vi "Remove Object.vi"(8 "error in (no error)":errorcluster, 10 "UUID":string, 11 "Controller in":refnum<class "Controller.lvclass">) -> (0 "error out":errorcluster, 3 "Controller out":refnum<class "Controller.lvclass">)   [LabVIEW 2013, in "SET Project Editor.lvlib" / "Controller.lvclass"]
uses:
  Controller.lvclass
  Controller.lvclass/Controller.ctl
  SET Project Data/Project Data Class/Project Data.lvclass
  SET Project Data/Menu Class/Menu Data.lvclass/Menu Data.ctl
  SET Project Data/VI Class/VI Data.lvclass
  SET Project Data/Control Classes/GObject/GObject.lvclass/GObject.ctl
  <vilib>/ActorFramework/Message Enqueuer/Message Enqueuer.lvclass/Message Enqueuer.ctl
  SET Project Data/Menu Class/Write Menu Item LUT.vi
  SET Project Data/Menu Class/Read Menu Item LUT.vi
  SET Project Data/Control Classes/GObject/Write Items.vi
  SET Project Data/Control Classes/GObject/Read Items.vi
  <vilib>/ActorFramework/Message Enqueuer/Enqueue.vi
  <vilib>/ActorFramework/Message Priority Queue/Priority Enqueue.vi
  UI View Messages/UI Refresh Data Msg/UI Refresh Data Msg.lvclass
  SET Project Editor.lvlib
  SET Project Data/Control Classes/GObject/GObject.lvclass
  SET Project Data/Menu Class/Menu Data.lvclass
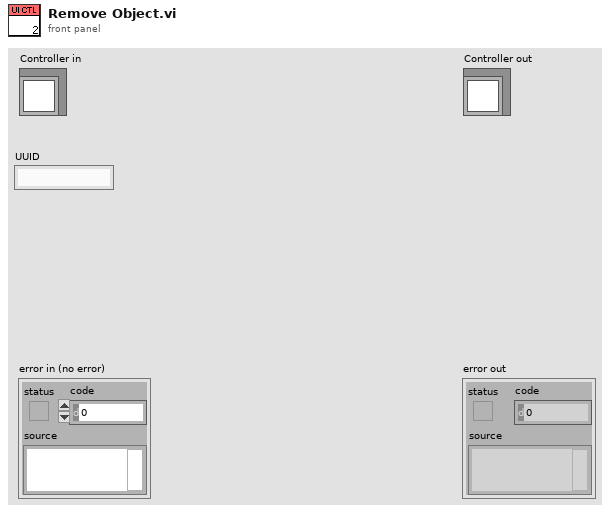
[diagram p1: front panel]
types:
  T1 = typedef "SET Project Editor.lvlib/UID Types.ctl" = enum16{"Invalid", "VI File", "GObject", "GObject Item", "RTM File", "RTM Item"}
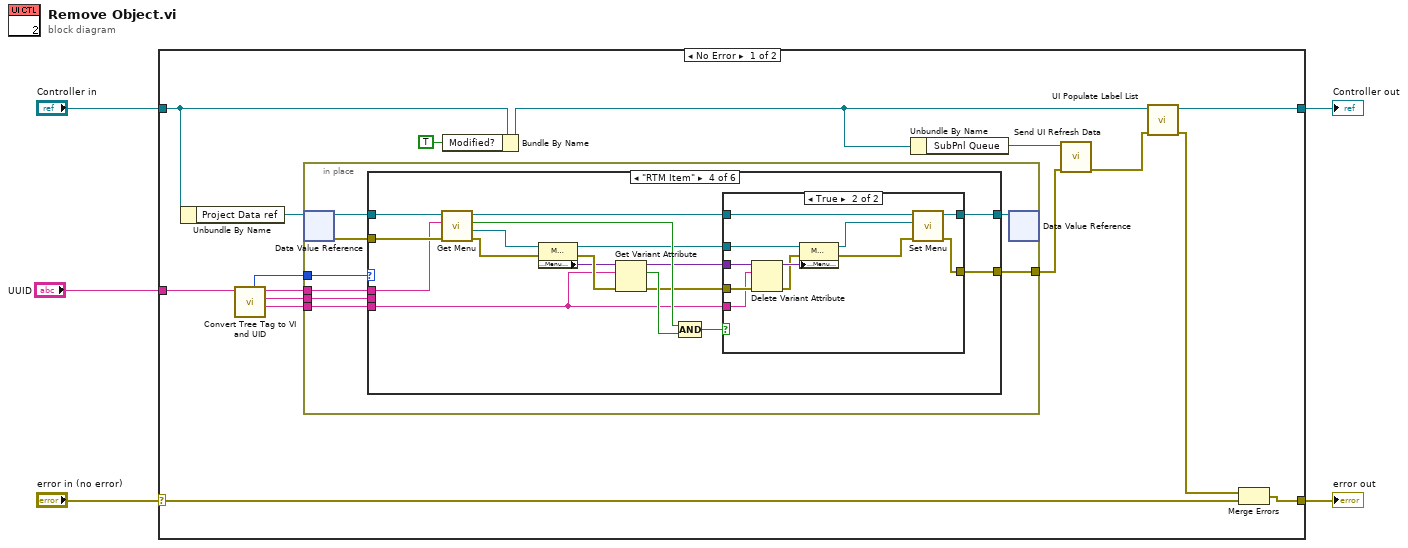
[diagram p0: block diagram]
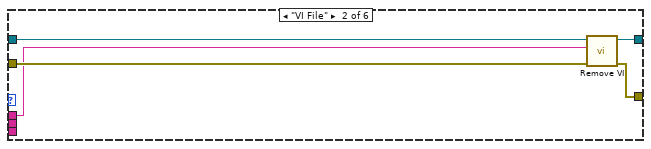
[diagram p3: hidden frame]
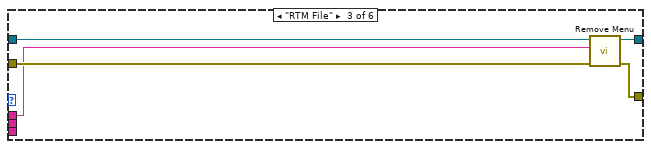
[diagram p4: hidden frame]
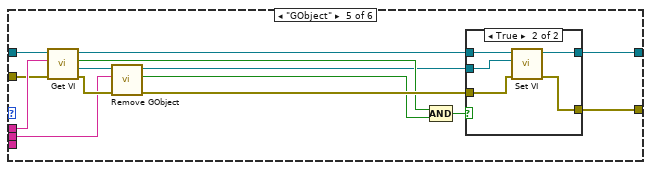
[diagram p6: hidden frame]
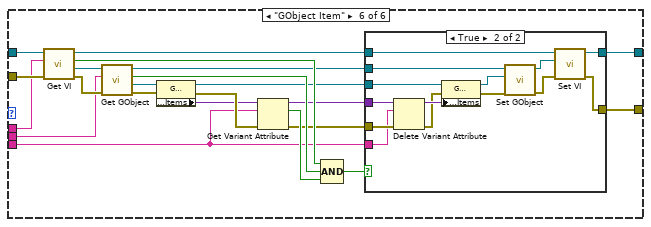
[diagram p8: hidden frame]
diagram:
  n1 = case shown="No Error" "error in (no error)" {
    selector: "error in (no error)" -> [w20 w132]
    tunnel: [w19 w132] -> w4
    tunnel: [w13 w131] -> w2
    tunnel: "Controller in" -> [w16 w131]
    tunnel: "UUID" -> [w10 _]
    frame No Error {
      n2 = Unbundle By Name(w16) -> ("Project Data ref"=w21:refnum<data-value>)
      n3 = call "Convert Tree Tag to VI and UID.vi"("Tree Tag"=w10) -> ("Item Name"=w6:string, "GObject UID"=w7:string, "File Path (Relative)"=w8:string, "UID Type"=w9:T1)  [unwired: 7 in]
      n4 = in-place {
        in-place-border: [w28] -> w17
        in-place-border: w9 -> [w25]
        in-place-border: w8 -> [w24]
        in-place-border: w7 -> [w23]
        in-place-border: w6 -> [w22]
        n5 = in-place-dvr #1(w21) -> (w27:refnum<class "Project Data.lvclass">, w26:errorcluster)
        n6 = case shown="\"RTM Item\"" w25 {
          tunnel: [w31 w35 w40 w46 w76 w97] -> w29
          tunnel: [w30 w33 w38 w42 w73 w96] -> w28
          tunnel: w27 -> [w31 w36 w41 w47 w77 w99]
          tunnel: w26 -> [w30 w34 w39 w45 w74 w98]
          tunnel: w24 -> [_ w32 w37 w44 w75 w95]
          tunnel: w23 -> [_ _ _ _ w72 w94]
          tunnel: w22 -> [_ _ _ w43 _ w93]
          frame "Invalid", Default {
          }
          frame "VI File" {
            n7 = call "Remove VI.vi"("error in (no error)"=w34, "VI Name"=w32, "ProjectData in"=w36) -> ("error out"=w33:errorcluster, "ProjectData out"=w35:refnum<class "Project Data.lvclass">)  [unwired: 5 in, 2 out]
          }
          frame "RTM File" {
            n8 = call "Remove Menu.vi"("error in (no error)"=w39, "Menu Name"=w37, "ProjectData in"=w41) -> ("error out"=w38:errorcluster, "ProjectData out"=w40:refnum<class "Project Data.lvclass">)  [unwired: 5 in, 2 out]
          }
          frame "RTM Item" {
            n9 = call-dynamic "Get Menu.vi"("error in (no error)"=w45, "Menu Path (Relative)"=w44, "ProjectData in"=w47) -> ("error out"=w58:errorcluster, "Menu Data out"=w57:refnum<class "Menu Data.lvclass">, "found"=w54:bool, "ProjectData out"=w48:refnum<class "Project Data.lvclass">)  [unwired: 5 in]
            n10 = property class="Menu Data.lvclass"(reference=w57, error in=w58) -> (reference out=w49:refnum<class "Menu Data.lvclass">, error out=w53:errorcluster, "Properties:Menu Item LUT"=w50:variant)
            n11 = Get Variant Attribute(Variant=w50, name=w43, error in=w53) -> (duplicate Variant=w51:variant, found=w55:bool, error out=w52:errorcluster)  [unwired: 1 in, 1 out]
            n12 = Compound Arithmetic op=AND(w54, w55) -> (w56:bool)
            n13 = case shown="True" w56 {
              tunnel: w48 -> [w60 w71]
              tunnel: [w60 w70] -> w46
              tunnel: w49 -> [_ w68]
              tunnel: [w59 w67] -> w42
              tunnel: w51 -> [_ w65]
              tunnel: w52 -> [w59 w64]
              tunnel: w43 -> [_ w63]
              frame False {
              }
              frame True {
                n14 = Delete Variant Attribute(4:w64, 6:w63, 7:w65) -> (0:w66:errorcluster, 3:w69:variant)  [unwired: 1 out]
                n15 = property class="Menu Data.lvclass"(reference=w68, error in=w66, "Properties:Menu Item LUT"=w69) -> (reference out=w62:refnum<class "Menu Data.lvclass">, error out=w61:errorcluster)
                n16 = call-dynamic "Set Menu.vi"("error in (no error)"=w61, "RTM Data in"=w62, "ProjectData in"=w71) -> ("error out"=w67:errorcluster, "ProjectData out"=w70:refnum<class "Project Data.lvclass">)  [unwired: 6 in, 1 out]
              }
            }
          }
          frame "GObject" {
            n17 = call-dynamic "Get VI.vi"("error in (no error)"=w74, "VI Path (Relative)"=w75, "ProjectData in"=w77) -> ("error out"=w80:errorcluster, "VI Data out"=w79:refnum<class "VI Data.lvclass">, "found"=w82:bool, "ProjectData out"=w78:refnum<class "Project Data.lvclass">)  [unwired: 5 in]
            n18 = call-dynamic "Remove GObject.vi"("error in (no error)"=w80, "GObject UID"=w72, "VI Data in"=w79) -> ("error out"=w85:errorcluster, "found"=w83:bool, "VI Data out"=w81:refnum<class "VI Data.lvclass">)  [unwired: 5 in, 1 out]
            n19 = Compound Arithmetic op=AND(w82, w83) -> (w84:bool)
            n20 = case shown="True" w84 {
              tunnel: w81 -> [_ w89]
              tunnel: w78 -> [w87 w92]
              tunnel: [w87 w91] -> w76
              tunnel: [w86 w90] -> w73
              tunnel: w85 -> [w86 w88]
              frame False {
              }
              frame True {
                n21 = call-dynamic "Set VI.vi"("error in (no error)"=w88, "VI Data in"=w89, "ProjectData in"=w92) -> ("error out"=w90:errorcluster, "ProjectData out"=w91:refnum<class "Project Data.lvclass">)  [unwired: 6 in, 1 out]
              }
            }
          }
          frame "GObject Item" {
            n22 = call-dynamic "Get VI.vi"("error in (no error)"=w98, "VI Path (Relative)"=w95, "ProjectData in"=w99) -> ("error out"=w101:errorcluster, "VI Data out"=w100:refnum<class "VI Data.lvclass">, "found"=w111:bool, "ProjectData out"=w103:refnum<class "Project Data.lvclass">)  [unwired: 5 in]
            n23 = call-dynamic "Get GObject.vi"("error in (no error)"=w101, "GObject UID"=w94, "VI Data in"=w100) -> ("error out"=w106:errorcluster, "GObject"=w104:refnum<class "GObject.lvclass">, "found"=w112:bool, "VI Data out"=w102:refnum<class "VI Data.lvclass">)  [unwired: 5 in]
            n24 = property class="GObject.lvclass"(reference=w104, error in=w106) -> (reference out=w105:refnum<class "GObject.lvclass">, error out=w110:errorcluster, "Properties:Items"=w107:variant)
            n25 = Get Variant Attribute(Variant=w107, name=w93, error in=w110) -> (duplicate Variant=w108:variant, found=w113:bool, error out=w109:errorcluster)  [unwired: 1 in, 1 out]
            n26 = Compound Arithmetic op=AND(w111, w112, w113) -> (w114:bool)
            n27 = case shown="True" w114 {
              tunnel: w102 -> [_ w130]
              tunnel: w103 -> [w116 w129]
              tunnel: [w116 w127] -> w97
              tunnel: w105 -> [_ w123]
              tunnel: [w115 w121] -> w96
              tunnel: w108 -> [_ w119]
              tunnel: w109 -> [w115 w118]
              tunnel: w93 -> [_ w117]
              frame False {
              }
              frame True {
                n28 = Delete Variant Attribute(4:w118, 6:w117, 7:w119) -> (0:w120:errorcluster, 3:w124:variant)  [unwired: 1 out]
                n29 = property class="GObject.lvclass"(reference=w123, error in=w120, "Properties:Items"=w124) -> (reference out=w126:refnum<class "GObject.lvclass">, error out=w125:errorcluster)
                n30 = call "Set GObject.vi"("error in (no error)"=w125, "GObject.lvclass"=w126, "VI Data in"=w130) -> ("error out"=w122:errorcluster, "VI Data out"=w128:refnum<class "VI Data.lvclass">)  [unwired: 6 in, 1 out]
                n31 = call-dynamic "Set VI.vi"("error in (no error)"=w122, "VI Data in"=w128, "ProjectData in"=w129) -> ("error out"=w121:errorcluster, "ProjectData out"=w127:refnum<class "Project Data.lvclass">)  [unwired: 6 in, 1 out]
              }
            }
          }
        }
        n32 = in-place-dvr #1(w29) -> ()  [unwired: 2 out]
      }
      n33 = Bundle By Name(cluster=w16, "Modified?"=TRUE) -> (w14:refnum<class "Controller.lvclass">)
      n34 = Unbundle By Name(w14) -> ("SubPnl Queue"=w18:refnum<class "Message Enqueuer.lvclass">)
      n35 = call "Send UI Refresh Data.vi"("error in (no error)"=w17, "Message Enqueuer"=w18) -> ("error out"=w12:errorcluster)  [unwired: 8 in, 1 out]
      n36 = call-dynamic "UI Populate Label List.vi"("error in (no error)"=w12, "Controller in"=w14) -> ("error out"=w11:errorcluster, "Controller out"=w13:refnum<class "Controller.lvclass">)  [unwired: 8 in]
      n37 = Merge Errors(w11, w20) -> (w19:errorcluster)
    }
    frame Error {
    }
  }
  "error out" <- w4
  "Controller out" <- w2
